vi "Set Arm Position.vi"(8 "RobotDriveDevRef 2":T1={"DevStatus"={"status"=FALSE, "code"=0, "source"=""}, "Motors[]"=[{"DeviceStatus"={"status"=FALSE, "code"=0, "source"=""}, "Type"=enum."PWM", "PWM"={"PWM Channel"=enum."PWM 3", "DeadBand"={"Name"="Victor SP", "maxPositivePwm"=1504, "minPositivePwm"=1005, "centerPwm"=1000, "maxNegativePwm"=995, "minNegativePwm"=497, "angularRange"=0}}, "CAN"={"Device Number"=0, "Control Mode"=enum."Percent VBus", "Semaphore"=refnum, "Max Vout"=0.0, "TalonSRX Control Mode"=enum."Percent VBus"}, "Invert"=TRUE}, {"DeviceStatus"={"status"=FALSE, "code"=0, "source"=""}, "Type"=enum."PWM", "PWM"={"PWM Channel"=enum."PWM 1", "DeadBand"={"Name"="Victor SP", "maxPositivePwm"=1504, "minPositivePwm"=1005, "centerPwm"=1000, "maxNegativePwm"=995, "minNegativePwm"=497, "angularRange"=0}}, "CAN"={"Device Number"=0, "Control Mode"=enum."Percent VBus", "Semaphore"=refnum, "Max Vout"=0.0, "TalonSRX Control Mode"=enum."Percent VBus"}, "Invert"=FALSE}, {"DeviceStatus"={"status"=FALSE, "code"=0, "source"=""}, "Type"=enum."PWM", "PWM"={"PWM Channel"=enum."PWM 4", "DeadBand"={"Name"="Victor SP", "maxPositivePwm"=1504, "minPositivePwm"=1005, "centerPwm"=1000, "maxNegativePwm"=995, "minNegativePwm"=497, "angularRange"=0}}, "CAN"={"Device Number"=0, "Control Mode"=enum."Percent VBus", "Semaphore"=refnum, "Max Vout"=0.0, "TalonSRX Control Mode"=enum."Percent VBus"}, "Invert"=TRUE}, {"DeviceStatus"={"status"=FALSE, "code"=0, "source"=""}, "Type"=enum."PWM", "PWM"={"PWM Channel"=enum."PWM 2", "DeadBand"={"Name"="Victor SP", "maxPositivePwm"=1504, "minPositivePwm"=1005, "centerPwm"=1000, "maxNegativePwm"=995, "minNegativePwm"=497, "angularRange"=0}}, "CAN"={"Device Number"=0, "Control Mode"=enum."Percent VBus", "Semaphore"=refnum, "Max Vout"=0.0, "TalonSRX Control Mode"=enum."Percent VBus"}, "Invert"=FALSE}], "Square Inputs"=TRUE, "Max Output"=1.0}, 10 "Speed":dbl=1.0, 11 "Setpoint":dbl=500.0) -> (0 "RobotDriveDevRef":T1={"DevStatus"={"status"=FALSE, "code"=0, "source"=""}, "Motors[]"=[{"DeviceStatus"={"status"=FALSE, "code"=0, "source"=""}, "Type"=enum."PWM", "PWM"={"PWM Channel"=enum."PWM 3", "DeadBand"={"Name"="Victor SP", "maxPositivePwm"=1504, "minPositivePwm"=1005, "centerPwm"=1000, "maxNegativePwm"=995, "minNegativePwm"=497, "angularRange"=0}}, "CAN"={"Device Number"=0, "Control Mode"=enum."Percent VBus", "Semaphore"=refnum, "Max Vout"=0.0, "TalonSRX Control Mode"=enum."Percent VBus"}, "Invert"=TRUE}, {"DeviceStatus"={"status"=FALSE, "code"=0, "source"=""}, "Type"=enum."PWM", "PWM"={"PWM Channel"=enum."PWM 1", "DeadBand"={"Name"="Victor SP", "maxPositivePwm"=1504, "minPositivePwm"=1005, "centerPwm"=1000, "maxNegativePwm"=995, "minNegativePwm"=497, "angularRange"=0}}, "CAN"={"Device Number"=0, "Control Mode"=enum."Percent VBus", "Semaphore"=refnum, "Max Vout"=0.0, "TalonSRX Control Mode"=enum."Percent VBus"}, "Invert"=FALSE}, {"DeviceStatus"={"status"=FALSE, "code"=0, "source"=""}, "Type"=enum."PWM", "PWM"={"PWM Channel"=enum."PWM 4", "DeadBand"={"Name"="Victor SP", "maxPositivePwm"=1504, "minPositivePwm"=1005, "centerPwm"=1000, "maxNegativePwm"=995, "minNegativePwm"=497, "angularRange"=0}}, "CAN"={"Device Number"=0, "Control Mode"=enum."Percent VBus", "Semaphore"=refnum, "Max Vout"=0.0, "TalonSRX Control Mode"=enum."Percent VBus"}, "Invert"=TRUE}, {"DeviceStatus"={"status"=FALSE, "code"=0, "source"=""}, "Type"=enum."PWM", "PWM"={"PWM Channel"=enum."PWM 2", "DeadBand"={"Name"="Victor SP", "maxPositivePwm"=1504, "minPositivePwm"=1005, "centerPwm"=1000, "maxNegativePwm"=995, "minNegativePwm"=497, "angularRange"=0}}, "CAN"={"Device Number"=0, "Control Mode"=enum."Percent VBus", "Semaphore"=refnum, "Max Vout"=0.0, "TalonSRX Control Mode"=enum."Percent VBus"}, "Invert"=FALSE}], "Square Inputs"=TRUE, "Max Output"=1.0})   [LabVIEW 2015]
uses:
  <vilib>/Rock Robotics/WPI/RobotDrive/WPI_RobotDriveDevRef.ctl
  <vilib>/Rock Robotics/WPI/MotorControl/WPI_MotorControlDeviceRef.ctl
  <vilib>/Rock Robotics/WPI/MotorControl/WPI_MotorControlType.ctl
  <vilib>/Rock Robotics/SystemInterfaces/DIO/FPGA_DIOPWMChannel.ctl
  <vilib>/Rock Robotics/WPI/PWM/WPI_PWMDeadband.ctl
  <vilib>/Rock Robotics/WPI/CAN/Jaguar/SubVIs/WPI_CANJaguar_ControlMode.ctl
  <vilib>/Rock Robotics/WPI/CAN/TalonSRX/WPI_CANTalonSRX_APIControlMode.ctl
  <vilib>/Rock Robotics/WPI/Utilities/WPI_GetSetVariantRefNum.vi
  Robot Global Data.vi
  <vilib>/addons/control/pid/pid.llb/PID (DBL).vi
  <vilib>/addons/control/pid/NI_PID_pid.lvlib
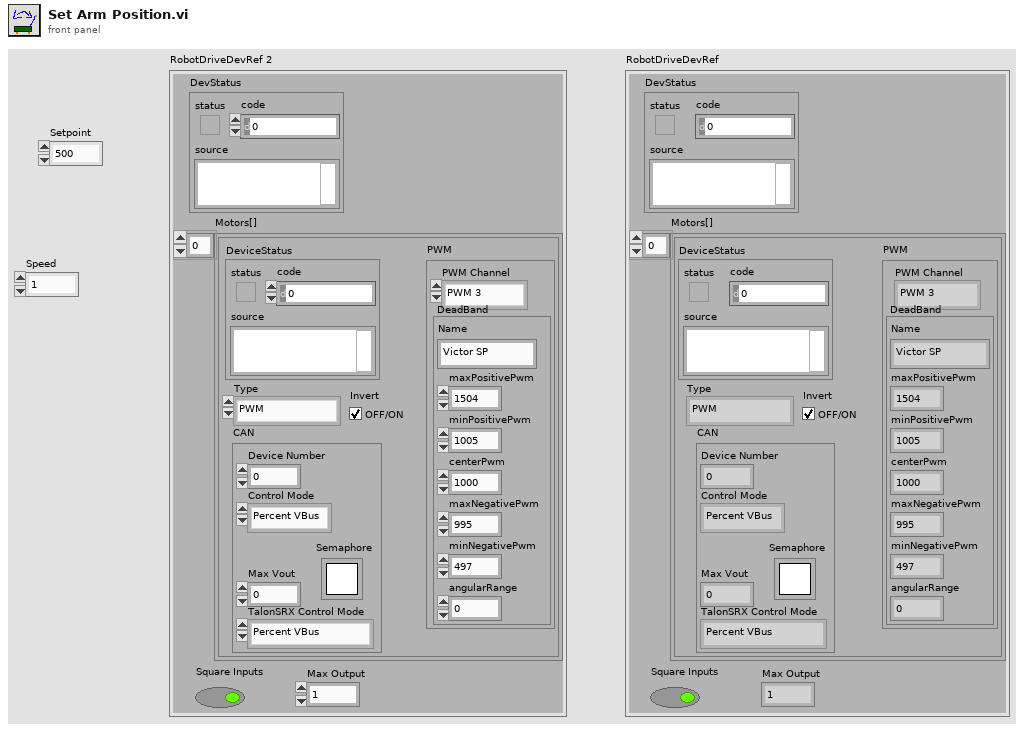
[diagram p1: front panel]
types:
  T1 = typedef "WPI_RobotDriveDevRef.ctl" = cluster{"DevStatus":errorcluster, "Motors[]":T2[], "Square Inputs":bool, "Max Output":dbl}
  T2 = typedef "WPI_MotorControlDeviceRef.ctl" = cluster{"DeviceStatus":errorcluster, "Type":T3, "PWM":cluster{"PWM Channel":T4, "DeadBand":T5}, "CAN":cluster{"Device Number":u8, "Control Mode":T6, "Semaphore":T7, "Max Vout":dbl, "TalonSRX Control Mode":T8}, "Invert":bool}
  T3 = typedef "WPI_MotorControlType.ctl" = enum16{"PWM", "CAN", "CANTalonSRX"}
  T4 = typedef "FPGA_DIOPWMChannel.ctl" = enum8{"PWM 0", "PWM 1", "PWM 2", "PWM 3", "PWM 4", "PWM 5", "PWM 6", "PWM 7", "PWM 8", "PWM 9", "PWM MXP 0", "PWM MXP 1", "PWM MXP 2", "PWM MXP 3", "PWM MXP 4", "PWM MXP 5", "PWM MXP 6", "PWM MXP 7", "PWM MXP 8", "PWM MXP 9", "Invalid"}
  T5 = typedef "WPI_PWMDeadband.ctl" = cluster{"Name":string, "maxPositivePwm":i32, "minPositivePwm":i32, "centerPwm":i32, "maxNegativePwm":i32, "minNegativePwm":i32, "angularRange":u16}
  T6 = typedef "WPI_CANJaguar_ControlMode.ctl" = enum8{"Percent VBus", "Current", "Speed", "Position", "Voltage"}
  T7 = typedef "Semaphore RefNum" = refnum<k1>
  T8 = typedef "WPI_CANTalonSRX_APIControlMode.ctl" = enum8{"Percent VBus", "Speed", "Position", "Slave", "Unchanged / Invalid", "Voltage Compensation", "Current", "Motion Profile"}
  T9 = typedef "WPI_SwitchDevRef.ctl" = cluster{"DevStatus":errorcluster, "DIO Channel":T10, "CntIndex":T11, "Normally Closed":bool}
  T10 = typedef "FPGA_DIOChannel.ctl" = enum8{"DIO 0", "DIO 1", "DIO 2", "DIO 3", "DIO 4", "DIO 5", "DIO 6", "DIO 7", "DIO 8", "DIO 9", "DIO MXP 0", "DIO MXP 1", "DIO MXP 2", "DIO MXP 3", "DIO MXP 4", "DIO MXP 5", "DIO MXP 6", "DIO MXP 7", "DIO MXP 8", "DIO MXP 9", "DIO MXP 10", "DIO MXP 11", "DIO MXP 12", "DIO MXP 13", "DIO MXP 14", "DIO MXP 15", "Invalid"}
  T11 = typedef "FPGA_CounterCtrSystemIndex.ctl" = enum8{"Ctr 0", "Ctr 1", "Ctr 2", "Ctr 3", "Ctr 4", "Ctr 5", "Ctr 6", "Ctr 7", "Invalid"}
  T12 = typedef "WPI_PotentiometerDevRef.ctl" = cluster{"DevStatus":errorcluster, "Analog Channel":T13, "Invert Output":bool}
  T13 = typedef "FPGA_AIChannel.ctl" = enum8{"AI 0", "AI 1", "AI 2", "AI 3", "AI MXP 0", "AI MXP 1", "AI MXP 2", "AI MXP 3", "Invalid"}
  T14 = cluster{"proportional gain (Kc)":dbl, "integral time (Ti, min)":dbl, "derivative time (Td, min)":dbl}
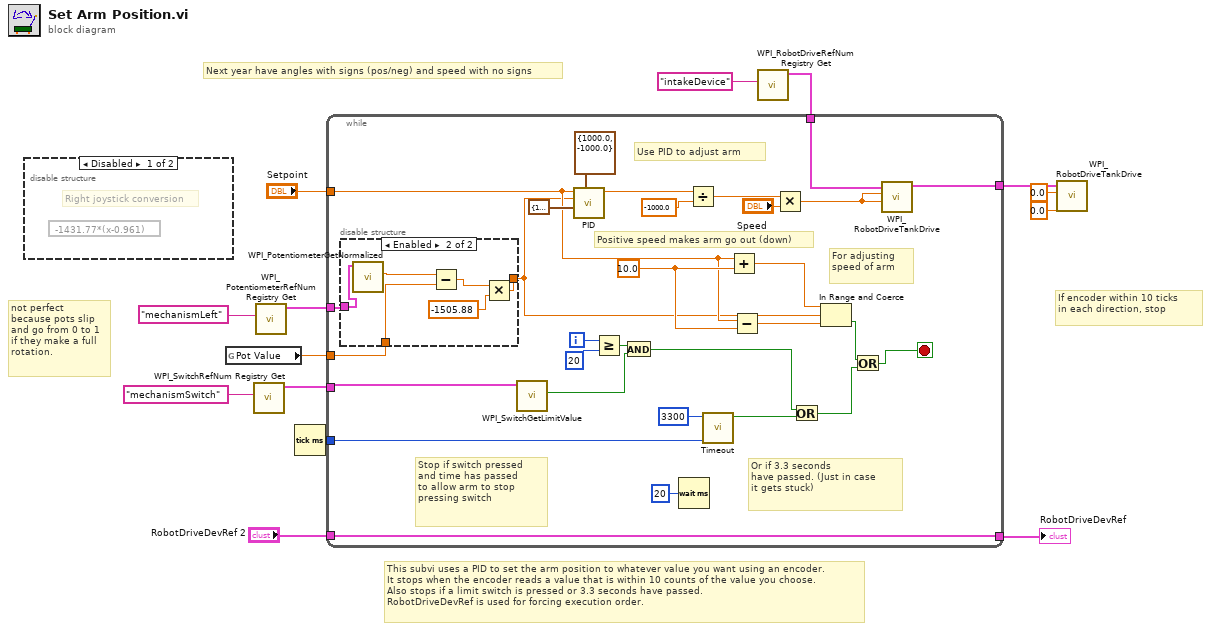
[diagram p0: block diagram]
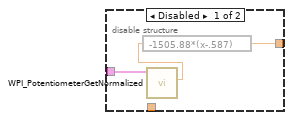
[diagram p3: hidden frame]
diagram:
  # "not perfect\nbecause pots slip\nand go from 0 to 1\nif they make a full\nrotation."
  # "Next year have angles with signs (pos/neg) and speed with no signs"
  # "If encoder within 10 ticks\nin each direction, stop"
  # "This subvi uses a PID to set the arm position to whatever value you want using an encoder.\nIt stops when the encoder reads a value that is within 10 counts of the value you choose.\nAlso stops if a limit switch is pressed or 3.3 seconds have passed.\nRobotDriveDevRef is used for forcing execution order."
  n1 = disable-structure shown="Disabled" {
    frame Disabled {
      # "Right joystick conversion"
      n2 = expression code="-1431.77*(x-0.961)"() -> ()  [unwired: 1 in, 1 out]
    }
    frame Enabled {
    }
  }
  n3 = global read "Robot Global Data.vi" "Pot Value"() -> (w4:dbl)
  n4 = call <vilib>:"WPI_SwitchRefNum Registry Get.vi"("refnum name"="mechanismSwitch") -> ("SwitchDevRef"=w6:T9)  [unwired: 9 in, 1 out]
  n5 = call <vilib>:"WPI_PotentiometerRefNum Registry Get.vi"("refnum name"="mechanismLeft") -> ("PotDevRef"=w13:T12)  [unwired: 9 in, 1 out]
  n6 = Tick Count (ms)() -> (millisecond timer value=w5:u32)
  n7 = call <vilib>:"WPI_RobotDriveRefNum Registry Get.vi"("refnum name"="intakeDevice") -> ("RobotDriveDevRef"=w8:T1)  [unwired: 9 in, 1 out]
  n8 = while {
    tunnel: w13 -> [w17]
    tunnel: "Setpoint" -> [w32]
    tunnel: "RobotDriveDevRef 2" -> [w38]
    tunnel: [w38] -> w10
    tunnel: w8 -> [w37]
    tunnel: w6 -> [w36]
    tunnel: w5 -> [w22]
    tunnel: w4 -> [w16]
    tunnel: [w15] -> w3
    i -> [w26]
    stop <- w34 stop-if-true
    w41 = 10.0 ("setpoint")
    # "Positive speed makes arm go out (down)"
    # "Stop if switch pressed\nand time has passed\nto allow arm to stop\npressing switch"
    # "Or if 3.3 seconds \nhave passed. (Just in case\nit gets stuck)"
    # "For adjusting \nspeed of arm"
    # "Use PID to adjust arm"
    n9 = disable-structure shown="Enabled" {
      disable-tunnel: w17 -> [w47 w49]
      disable-tunnel: [w46 w50] -> w18
      disable-tunnel: w16 -> [_ w48]
      frame Disabled {
        n10 = call <vilib>:"WPI_PotentiometerGetNormalized.vi"("PotDevRef"=w47) -> ("Normalized Value"=w45:dbl)  [unwired: 8 in, 2 out]
        n11 = expression code="-1505.88*(x-.587)"(w45) -> (w46:dbl)
      }
      frame Enabled {
        n12 = call <vilib>:"WPI_PotentiometerGetNormalized.vi"("PotDevRef"=w49) -> ("Normalized Value"=w51:dbl)  [unwired: 8 in, 2 out]
        n13 = Subtract(x=w51, y=w48) -> (x-y=w52:dbl)
        n14 = Multiply(x=w52, y=-1505.88) -> (x*y=w50:dbl)
      }
    }
    n15 = call <vilib>:"WPI_SwitchGetLimitValue.vi"("SwitchDevRef"=w36) -> ("Switch Pressed"=w21:bool)  [unwired: 8 in, 2 out]
    n16 = call-poly <vilib>:"PID.vi"("output range"=cluster{"output high":dbl, "output low":dbl} {"output high"=1000.0, "output low"=-1000.0}, "PID gains"=T14 {"proportional gain (Kc)"=1.0, "integral time (Ti, min)"=0.005, "derivative time (Td, min)"=0.0}, "process variable"=w18, "setpoint"=w32) -> ("output"=w31:dbl)  [unwired: 6 in, 1 out]
    n17 = Greater Or Equal?(x=w26, y=20) -> (x >= y?=w20:bool)
    n18 = And(x=w20, y=w21) -> (x .and. y?=w25:bool)
    n19 = Wait (ms)(milliseconds to wait=u32 20) -> ()  [unwired: 1 out]
    n20 = Divide(x=w31, y=-1000.0) -> (x/y=w29:dbl)
    n21 = call "Timeout.vi"("Start Time In"=w22, "Time Limit"=u32 3300) -> ("Timeout"=w23:bool)  [unwired: 8 in, 1 out]
    n22 = Add(x=w32, y=w41) -> (x+y=w39:dbl)
    n23 = Subtract(x=w32, y=w41) -> (x-y=w40:dbl)
    n24 = Multiply(x=w29, y="Speed") -> (x*y=w19:dbl)
    n25 = Or(x=w25, y=w23) -> (x .or. y?=w30:bool)
    n26 = In Range and Coerce(upper limit=w39, x=w18, lower limit=w40) -> (In Range?=w35:bool)  [unwired: 1 out]
    n27 = Or(x=w35, y=w30) -> (x .or. y?=w34:bool)
    n28 = call <vilib>:"WPI_RobotDriveTankDrive.vi"("Right axis value"=w19, "Left axis value"=w19, "RobotDriveDevRef"=w37) -> ("RobotDriveDevRef"=w15:T1)  [unwired: 6 in, 2 out]
  }
  "RobotDriveDevRef" <- w10
  n29 = call <vilib>:"WPI_RobotDriveTankDrive.vi"("Right axis value"=0.0, "Left axis value"=0.0, "RobotDriveDevRef"=w3) -> ()  [unwired: 6 in, 3 out]
